vi "Vision Target Values.vi"() -> ()   [LabVIEW 2015]
panel:
  out "Vision target values":T1 {"Detected Targets"."Normalized Rect"."Numeric 5" format="%#_2g"; "Detected Targets"."Normalized Rect"."Numeric 3" format="%#_2g"; "Detected Targets"."Normalized Rect"."Numeric 2" format="%#_2g"; "Detected Targets"."Normalized Rect"."Numeric" format="%#_2g"}
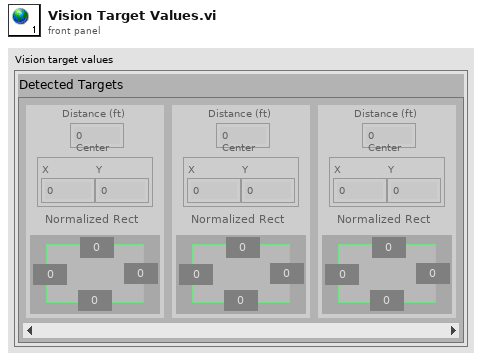
[diagram p1: front panel]
types:
  T1 = cluster{"Detected Targets":cluster{"Distance (ft)":dbl, "Center":cluster{"X":dbl, "Y":dbl}, "Normalized Rect":cluster{"Numeric":dbl, "Numeric 2":dbl, "Numeric 3":dbl, "Numeric 5":dbl}}[]}
diagram:
